vi "svl_Decimation with IC (Resampled).vi"(6 "new dr":dbl, 8 "initial decimation state":i32, 9 "init/cont (init:F)":bool, 10 "decimating factor (1)":i32=1 min=1 step=1, 11 "even angle signal":T1 {"even angle signal" format="%.2f"; "dr" format="%.2f"; "r0" format="%.2f"}) -> (0 "final decimation state":i32, 3 "even angle signal":T1 {"even angle signal" format="%.2f"; "dr" format="%.2f"; "r0" format="%.2f"})   [LabVIEW 2017]
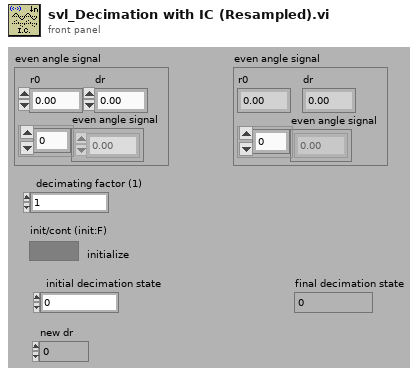
[diagram p1: front panel]
types:
  T1 = cluster{"r0":dbl, "dr":dbl, "even angle signal":dbl[]}
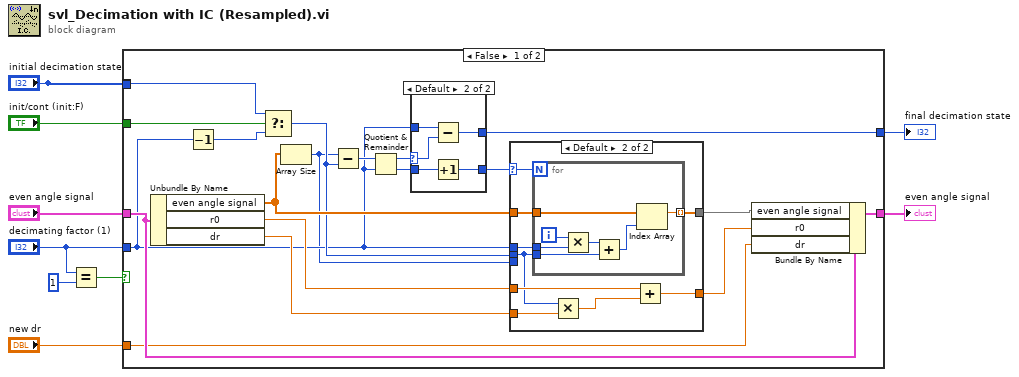
[diagram p0: block diagram]
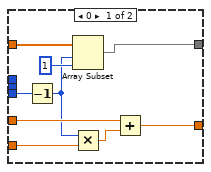
[diagram p2: hidden frame]
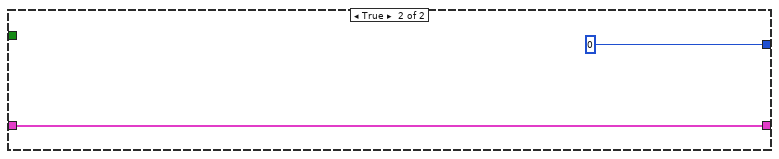
[diagram p4: hidden frame]
diagram:
  n1 = Equal?(x="decimating factor (1)", y=1) -> (x = y?=w5:bool)
  n2 = case shown="False" w5 {
    tunnel: [w20 w62] -> w9
    tunnel: "even angle signal" -> [w22 w62]
    tunnel: "initial decimation state" -> [_ _]
    tunnel: "decimating factor (1)" -> [w13 _]
    tunnel: [w26 0] -> w4
    tunnel: "init/cont (init:F)" -> [w25 _]
    tunnel: "initial decimation state" -> [w24 _]
    tunnel: "new dr" -> [w19 _]
    frame False {
      n3 = Unbundle By Name(w22) -> ("even angle signal"=w23:dbl[], "r0"=w18:dbl, "dr"=w17:dbl)
      n4 = Decrement(x=w13) -> (x-1=w14:i32)
      n5 = Select(t=w24, s=w25, f=w14) -> (s? t:f=w16:i32)
      n6 = Array Size(array=w23) -> (size(s)=w10:i32)
      n7 = Subtract(x=w10, y=w16) -> (x-y=w28:i32)
      n8 = Quotient & Remainder(x=w28, y=w13) -> (x-y*floor(x/y)=w12:i32, floor(x/y)=w27:i32)
      n9 = case shown="Default" w12 {
        selector: w12 -> [w54 w56]
        tunnel: w27 -> [w55 w60]
        tunnel: [w55 w59] -> w11
        tunnel: [w54 w57] -> w26
        tunnel: w13 -> [_ w58]
        frame 0 {
        }
        frame Default {
          n10 = Subtract(x=w58, y=w56) -> (x-y=w57:i32)
          n11 = Increment(x=w60) -> (x+1=w59:i32)
        }
      }
      n12 = case shown="Default" w11 {
        selector: w11 -> [_ w39]
        tunnel: w23 -> [w36 w46]
        tunnel: [w30 w45] -> w21
        tunnel: w18 -> [w34 w43]
        tunnel: w17 -> [w32 w42]
        tunnel: w16 -> [_ w38]
        tunnel: [w29 w41] -> w15
        tunnel: w13 -> [_ w40]
        tunnel: w10 -> [w37 _]
        frame 0 {
          n13 = Decrement(x=w37) -> (x-1=w33:i32)
          n14 = Array Subset(array=w36, index=w33, length=1) -> (w30:dbl[])
          n15 = Multiply(x=w33, y=w32) -> (x*y=w31:dbl)
          n16 = Add(x=w34, y=w31) -> (x+y=w29:dbl)
        }
        frame Default {
          n17 = for {
            N: w39 -> [_]
            tunnel: w40 -> [w52]
            tunnel: w46 -> [w53]
            tunnel: w38 -> [w48]
            tunnel: [w47] -> w45 mode=indexing
            i -> [w51]
            n18 = Multiply(x=w51, y=w52) -> (x*y=w50:i32)
            n19 = Add(x=w50, y=w48) -> (x+y=w49:i32)
            n20 = Index Array(array=w53, index=w49) -> (element=w47:dbl)
          }
          n21 = Multiply(x=w38, y=w42) -> (x*y=w44:dbl)
          n22 = Add(x=w43, y=w44) -> (x+y=w41:dbl)
        }
      }
      n23 = Bundle By Name(cluster=w22, "even angle signal"=w21, "r0"=w15, "dr"=w19) -> (w20:T1)
    }
    frame True {
    }
  }
  "even angle signal" <- w9
  "final decimation state" <- w4
